vi "Insert Halt.vi"(6 "Insertion Index":i32=-1, 7 "Parent ID":string, 8 "error in (no error)":errorcluster, 9 "Unique ID":string, 10 "Name":string, 11 "Test Executive in":refnum<class "Test Executive.lvclass">) -> (0 "error out":errorcluster, 1 "Replaced?":bool, 3 "Test Executive out":refnum<class "Test Executive.lvclass">, 5 "Unique ID out":string)   [LabVIEW 2017, in "Test Executive.lvlib" / "Test Executive.lvclass"]
uses:
  <vilib>/gpm_packages/@cs/test-executive/Source/Test Executive/TestExecutive/Test Executive.lvclass
  <vilib>/gpm_packages/@cs/test-executive/Source/Test Executive/Halt/Halt.lvclass
  <vilib>/gpm_packages/@cs/test-executive/Source/Test Executive/TestExecutive/Test Executive.lvclass/Test Executive.ctl
  <vilib>/gpm_packages/@cs/linked-list/Source/Linked List/Linked List Ref/Linked List Ref.lvclass
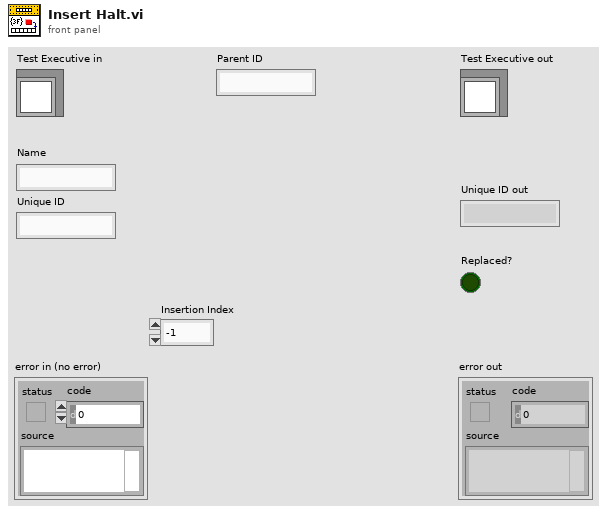
[diagram p1: front panel]
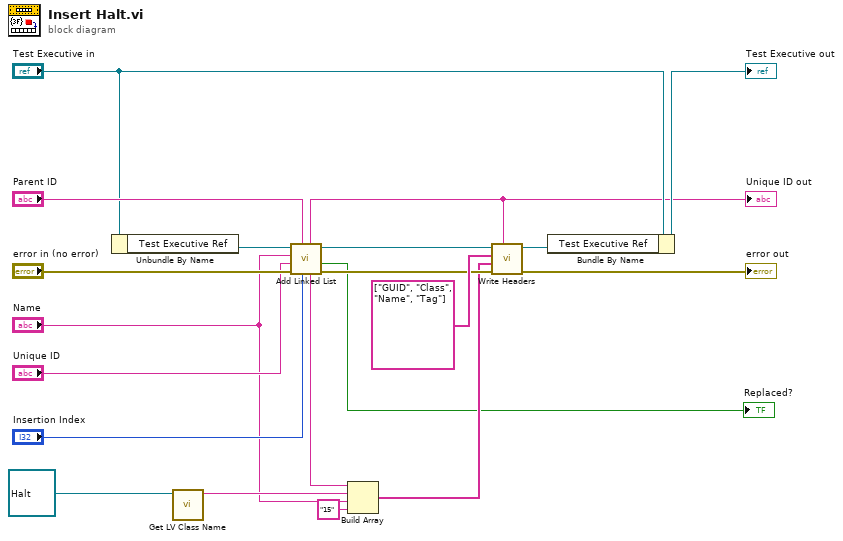
[diagram p0: block diagram]
diagram:
  n1 = Unbundle By Name("Test Executive in") -> ("Test Executive Ref"=w15:refnum<data-value>)
  n2 = call <vilib>:"Get LV Class Name.vi"("object"=refnum<class "Halt.lvclass"> refnum ("Test Executive.lvlib:Halt.lvclass")) -> ("class name"=w12:string)  [unwired: 9 in, 1 out]
  n3 = call <vilib>:"Add Linked List.vi"("Insertion Index"="Insertion Index", "Parent ID"="Parent ID", "error in (no error)"="error in (no error)", "Linked List ID"="Unique ID", "Name"="Name", "Linked List Ref"=w15) -> ("error out"=w17:errorcluster, "Replaced?"=→"Replaced?":bool, "Linked List Ref out"=w14:refnum<data-value>, "Linked List ID out"=w5:string)  [unwired: 2 in]
  "Unique ID out" <- w5
  n4 = Build Array(w5, w12, "Name", "15" ("element")) -> (w16:string[])
  n5 = call <vilib>:"Write Headers.vi"("Linked List ID"=w5, "error in (no error)"=w17, "Header Values"=w16, "Header Names"=string[] ["GUID", "Class", "Name", "Tag"], "Linked List Ref"=w14) -> ("error out"=→"error out":errorcluster, "Linked List Ref out"=w4:refnum<data-value>)  [unwired: 5 in]
  n6 = Bundle By Name(cluster="Test Executive in", "Test Executive Ref"=w4) -> (→"Test Executive out":refnum<class "Test Executive.lvclass">)
